vi "SPAN_Gasteiler_Endpunkt.vi"(11 "Komponente":i32) -> ()   [LabVIEW 2020, in "Linearisierung v2.lvlib" / "SpanEinstellungen.lvlib"]
uses:
  SpanEinstellungen.lvlib
  Gasteiler/Aktionen FGV Gasteiler Daten.ctl
  Aktion Lin Daten aufarbeiten.ctl
  Gasteiler/AK-Komm Gasteiler/Aktionen AK Komm.ctl
  Gasteiler/AK-Komm Gasteiler/Alter Gasteiler/Aktionen AK Komm_ALT.ctl
  Gasteiler/Horiba/Aktion Befehl.ctl
  Gasteiler/AK-Komm Gasteiler/AK Komm Gasteiler.lvlib
  Gasteiler/Horiba/Horiba GDC.lvlib
  Gasteiler/AK-Komm Gasteiler/Alter Gasteiler/Alter Gasteiler.lvlib
  Gasteiler/Gasteiler.lvlib
  Gasteiler/HovaCAL_Interface/Kommunikation/Kommunikation.lvlib
  Linearisierung v2.lvlib
  Gasteiler/HovaCAL_Interface/HovaCAL_Interface.lvlib
  Gasteiler/HovaCAL_Interface/Helper/Helper.lvlib
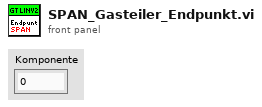
[diagram p1: front panel]
types:
  T1 = typedef "Linearisierung v2.lvlib/Aktion Lin Daten aufarbeiten.ctl" = enum16{"lesen", "Protkolldaten", "speichern", "laden", "EPA auswerten", "Tabelle schreiben", "Lin auswerten", "Tab init", "Stufentabelle", "EPA aktiviert", "Nachbehandlung laden", "Tabelle löschen", "Istwerte löschen", "Zeile löschen", "Zeile einfügen", "LIN aktiviert", "LIN/EPA aktiv laden", "EGAK Tab", "LIN übernehmen", "Tab init ohne Stufen"}
  T2 = typedef "Linearisierung v2.lvlib/Gasteiler.lvlib/Aktionen FGV Gasteiler Daten.ctl" = enum16{"lesen", "Gasteiler Daten", "Seriellen Param.", "MB-Endwert", "laden", "speichern", "Anforderung", "TCP", "Aufzeichnung Start"}
  T3 = typedef "Linearisierung v2.lvlib/Gasteiler.lvlib/Stufen Tabelle.ctl" = string[][]
  T4 = typedef "Linearisierung v2.lvlib/Lin-Polynom Daten.ctl" = cluster{"Messgerät":string, "Kalibrator (Gasteiler)":string, "Bearbeiter/in":string, "Komponente":string, "Zeitstempel":timestamp, "F_max gefordert (%)":sgl, "F_max in %":sgl, "F_max in ppm":sgl, "Vorschlag Ordnung":i32, "Polynom OK":bool, "Polynomkoeff.":dbl[], "Prüfgas Konzentration":dbl, "Pfad EPA":string, "Pfad_LIN":string, "Gasnummer:":u8, "Komponentenauswahl":T5, "Verdünnungsgas":T7, "Zeitdauer Stufe":T8, "Anzahl Stufen":T8, "F_max in % EPA":sgl, "F_max in ppm EPA":sgl, "F_max in % LIN":sgl, "F_max in ppm LIN":sgl, "Punkte umkehren":bool, "EPA Optionsfeld":T9, "Autolin Hovacal":T10, "Spanfactors":sgl[], "Kalibrierauswahl":T11, "Conditions:":T12, "Gasflaschen Nr.:":string, "Bottle Accuracy":dbl, "Konfig Gasflasche":T13, "Gasflasche":T14, "HovaCAL Flow AutoLin":T15, "MFC Output":T16, "Gas Ablaufdatum":timestamp, "Lin Modus":T17, "zusätzliche Zeitdauer Erster Punkt":sgl, "Offsets":sgl[]}
  T5 = typedef "Linearisierung v2.lvlib/KomponentenArray.ctl" = cluster{"Komponente:":T6, "Konzentration":dbl}[]
  T6 = typedef "Auswahlfeld.ctl" = u16
  T7 = typedef "Linearisierung v2.lvlib/Gasteiler.lvlib/Prüfgas in.ctl" = u16
  T8 = typedef "Zahlen-Eingabefeld.ctl" = sgl
  T9 = typedef "Linearisierung v2.lvlib/EPA Optionsfeld.ctl" = enum32{"Istwert", "Rohwert", "Linearisierter Wert"}
  T10 = typedef "Linearisierung v2.lvlib/Gasteiler.lvlib/HovaCal.lvlib/AutoLin Hovacal.ctl" = enum32{"Keine Auswahl", "Optionsauswahl 1", "Optionsauswahl 2"}
  T11 = typedef "Linearisierung v2.lvlib/Kalibrieroption.ctl" = u16
  T12 = typedef "Linearisierung v2.lvlib/Linearity verification 1065-307.lvlib/Condition.ctl" = u16
  T13 = typedef "System Einstellungen V2.lvlib/Konfig Gasflasche.ctl" = bool
  T14 = typedef "System Einstellungen V2.lvlib/Gasflasche Auswahl.ctl" = u16
  T15 = typedef "Linearisierung v2.lvlib/Gasteiler.lvlib/HovaCAL_Interface.lvlib/Controls.lvlib/Flow Einstellung.ctl" = cluster{"HovaCAL Flow Input Cluster":dbl}
  T16 = typedef "Linearisierung v2.lvlib/Gasteiler.lvlib/HovaCAL_Interface.lvlib/Controls.lvlib/Pump state.ctl" = cluster{"Run":bool}
  T17 = typedef "CalGas Aufschaltung.lvlib/Lin Modus.ctl" = u16
  T18 = typedef "Linearisierung v2.lvlib/Gasteiler.lvlib/Gasteiler Daten.ctl" = cluster{"Gasteiler":T19, "Gasteiler Stufen":T20, "Gasteiler Type":T21, "Konfig Gasteiler":T22, "Gasteiler Span Eingänge":u16}
  T19 = typedef "String - Eingabefeld.ctl" = string
  T20 = typedef "Linearisierung v2.lvlib/Gasteiler.lvlib/Gasteiler Stufen.ctl" = u16
  T21 = typedef "Linearisierung v2.lvlib/GasteilerType.ctl" = u16
  T22 = typedef "System Einstellungen V2.lvlib/Gasteiler Auswahl.ctl" = u16
  T23 = typedef "Linearisierung v2.lvlib/Gasteiler.lvlib/AK Komm Gasteiler.lvlib/Aktionen AK Komm.ctl" = enum16{"lesen", "initialisieren", "beenden", "Status", "SMAN", "SREM", "STBY", "ASTF", "ASTZ", "SLST", "AGAT", "EGAK", "AGAK", "AKAK", "ADRU", "SKOP", "SVSA", "SVSZ", "SONO", "SAIR", "SNOX", "ANOX", "SSPL", "SRUC", "SLIN", "ALST", "ETYP", "SVIO", "LCYL", "CCYL", "DCYL", "SCYL", "GCYL", "DRGV", "DRDC"}
  T24 = typedef "Linearisierung v2.lvlib/Gasteiler.lvlib/AK Komm Gasteiler.lvlib/Alter Gasteiler.lvlib/Aktionen AK Komm_ALT.ctl" = enum16{"lesen", "initialisieren", "beenden", "SRES", "STBY", "SREM", "SMAN", "SLIN", "SLCH", "SLST", "SSPL", "AGAT", "ALST", "ASTZ", "ASTF", "AGAK", "EGAK"}
  T25 = typedef "Linearisierung v2.lvlib/Gasteiler.lvlib/Horiba GDC.lvlib/Aktion Befehl.ctl" = enum16{"lesen", "initialisieren", "Beenden", "Standby", "GD/CC", "Info", "Flow", "Alarm", "GD parameter", "GD point", "Durchfluss", "Spuelen1", "Spuelen1 On", "Spuelen1Off", "Spuelen2", "Ventil-Abfrage", "Reset"}
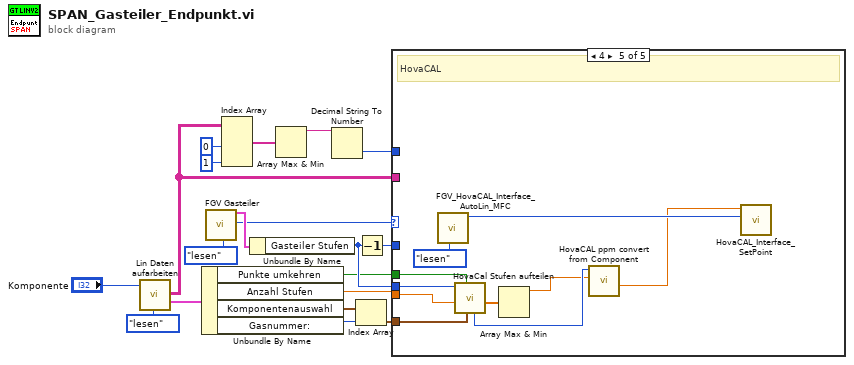
[diagram p0: block diagram]
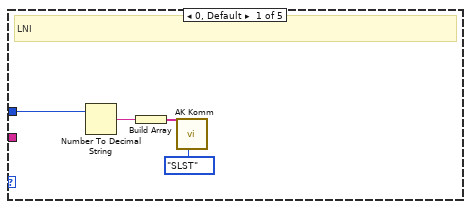
[diagram p2: hidden frame]
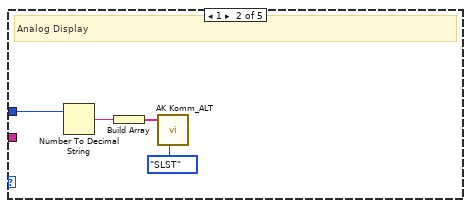
[diagram p3: hidden frame]
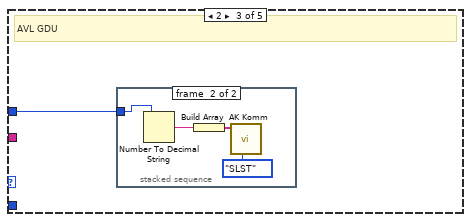
[diagram p4: hidden frame]
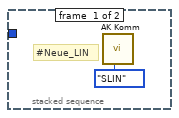
[diagram p5: hidden frame]
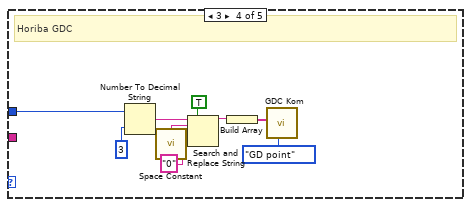
[diagram p6: hidden frame]
diagram:
  n1 = call "Lin Daten aufarbeiten.vi"("Index (Seite)"="Komponente", "Aktionen"=Aktion_Lin_Daten_aufarbeiten."lesen") -> ("Stufen Tabelle"=w6:T3, "Lin-Polynom"=w14:T4)  [unwired: 15 in, 9 out]
  n2 = Unbundle By Name(w14) -> ("Punkte umkehren"=w8:bool, "Anzahl Stufen"=w9:T8, "Komponentenauswahl"=w13:T5, "Gasnummer:"=w12:u8)
  n3 = call "FGV Gasteiler.vi"("Aktionen"=Aktionen_FGV_Gasteiler_Daten."lesen") -> ("Gasteiler Daten"=w18:T18, "Gasteiler Type"=w16:T21)  [unwired: 11 in, 6 out]
  n4 = Index Array(array=w6, index (col) #1=0 ("Index (Zeile)"), index (col) #2=1 ("Index (Spalte)")) -> (element #1=w2:string[])  [unwired: 2 in, 1 out]
  n5 = Unbundle By Name(w18) -> ("Gasteiler Stufen"=w10:T20)
  n6 = Array Max & Min(array=w2) -> (max value=w3:string)  [unwired: 3 out]
  n7 = Decimal String To Number(string=w3) -> (number=w1:i32)  [unwired: 2 in, 1 out]
  n8 = Index Array(array=w13, index=w12) -> (element=w11:cluster{"Komponente:":T6, "Konzentration":dbl})
  n9 = Decrement(x=w10) -> (x-1=w19:T20)
  n10 = case shown="4" w16 {
    tunnel: w19 -> [_ _ _ _ _]
    tunnel: w11 -> [_ _ _ _ w51]
    tunnel: w10 -> [_ _ _ _ w50]
    tunnel: w9 -> [_ _ _ _ w49]
    tunnel: w8 -> [_ _ _ _ w48]
    tunnel: w6 -> [_ _ _ _ _]
    tunnel: w1 -> [w20 w24 w28 w34 _]
    frame 0, Default {
      # "LNI"
      n11 = Number To Decimal String(number=w20) -> (decimal integer string=w23:string)  [unwired: 1 in]
      n12 = Build Array(w23) -> (w22:string[])
      n13 = call "AK Komm.vi"("Aktionen"=Aktionen_AK_Komm."SLST", "Daten"=w22) -> ()  [unwired: 3 in, 7 out]
    }
    frame 1 {
      # "Analog Display"
      n14 = Number To Decimal String(number=w24) -> (decimal integer string=w27:string)  [unwired: 1 in]
      n15 = Build Array(w27) -> (w26:string[])
      n16 = call "AK Komm_ALT.vi"("Aktionen_ALT"=Aktionen_AK_Komm_ALT."SLST", "Daten"=w26) -> ()  [unwired: 5 in, 5 out]
    }
    frame 2 {
      # "AVL GDU"
      n17 = stacked-sequence {
        tunnel: w28 -> [_ w32]
        frame #0 {
          # "#Neue_LIN"
          n18 = call "AK Komm.vi"("Aktionen"=Aktionen_AK_Komm."SLIN") -> ()  [unwired: 4 in, 7 out]
        }
        frame #1 {
          n19 = Number To Decimal String(number=w32) -> (decimal integer string=w33:string)  [unwired: 1 in]
          n20 = Build Array(w33) -> (w31:string[])
          n21 = call "AK Komm.vi"("Aktionen"=Aktionen_AK_Komm."SLST", "Daten"=w31) -> ()  [unwired: 3 in, 7 out]
        }
      }
    }
    frame 3 {
      # "Horiba GDC"
      n22 = Number To Decimal String(number=w34, width (-)=i16 3 ("Breite (-)")) -> (decimal integer string=w36:string)
      n23 = call <vilib>:"Space Constant.vi"() -> ("String"=w40:string)
      n24 = Search and Replace String(replace all?=TRUE ("Alle ersetzen? (F)"), input string=w36, search string=w40, replace string="0" ("Ersetzungs-String (\"\")")) -> (result string=w37:string)  [unwired: 4 in, 3 out]
      n25 = Build Array(w37) -> (w41:string[])
      n26 = call "GDC Kom.vi"("Befehl"=Aktion_Befehl."GD point", "Daten"=w41) -> ()  [unwired: 3 in, 7 out]
    }
    frame 4 {
      # "HovaCAL"
      n27 = call "FGV_HovaCAL_Interface_AutoLin_MFC.vi"("Aktion"=enum16{"lesen", "schreiben"}."lesen") -> ("AutoLin MFC out"=w46:u16)  [unwired: 7 in, 3 out]
      n28 = call "HovaCal Stufen aufteilen.vi"("Komponentenauswahl"=w51, "Punkte umkehren"=w48, "Anzahl Stufen"=w49, "Gasteiler Stufen"=w50) -> ("Stufen"=w47:dbl[], "Komponente:"=w45:T6)  [unwired: 4 in, 2 out]
      n29 = Array Max & Min(array=w47) -> (max value=w44:dbl)  [unwired: 3 out]
      n30 = call "HovaCAL ppm convert from Component.vi"("Konzentration"=w44, "Gasnummer"=w45) -> ("Konzentration in ppm"=w43:dbl)  [unwired: 5 in, 4 out]
      n31 = call "HovaCAL_Interface_SetPoint.vi"("AutoLin MFC Index"=w46, "Konzentration"=w43) -> ()  [unwired: 9 in, 1 out]
    }
  }
